vi "9.1.vi"() -> ()   [LabVIEW 2020]
panel:
  in  "module path 3":path=path "C:/Users/Oliver/Videos/ylesanne2.py"
  in  "Cluster":T1
  in  "Numeric 2":i32
  in  "Folat 2":dbl
  out "Waveform Graph":T1(graph)
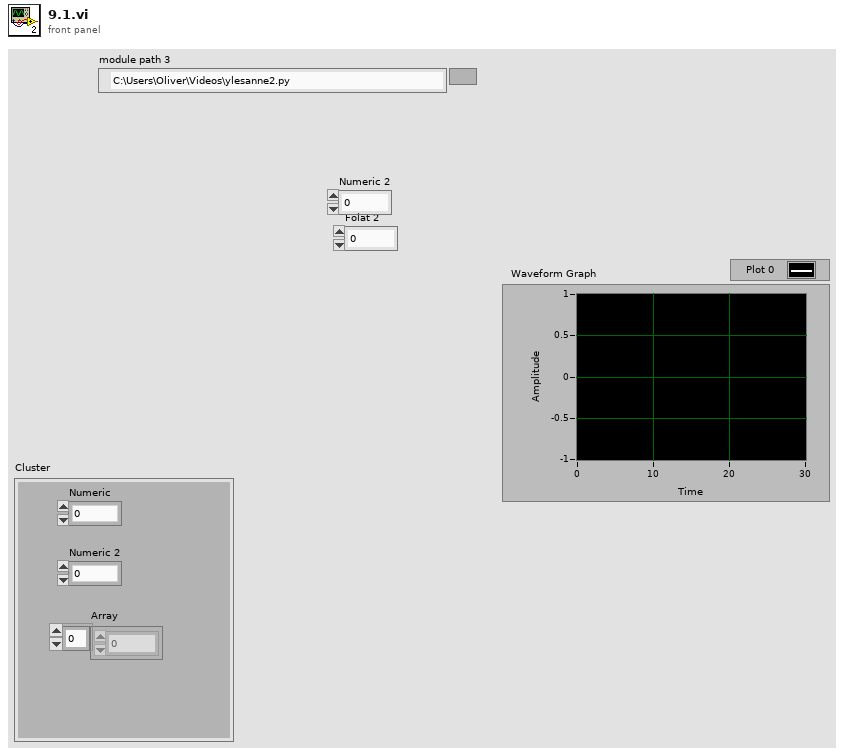
[diagram p1: front panel]
types:
  T1 = cluster{"Numeric":dbl, "Numeric 2":dbl, "Array":dbl[]}
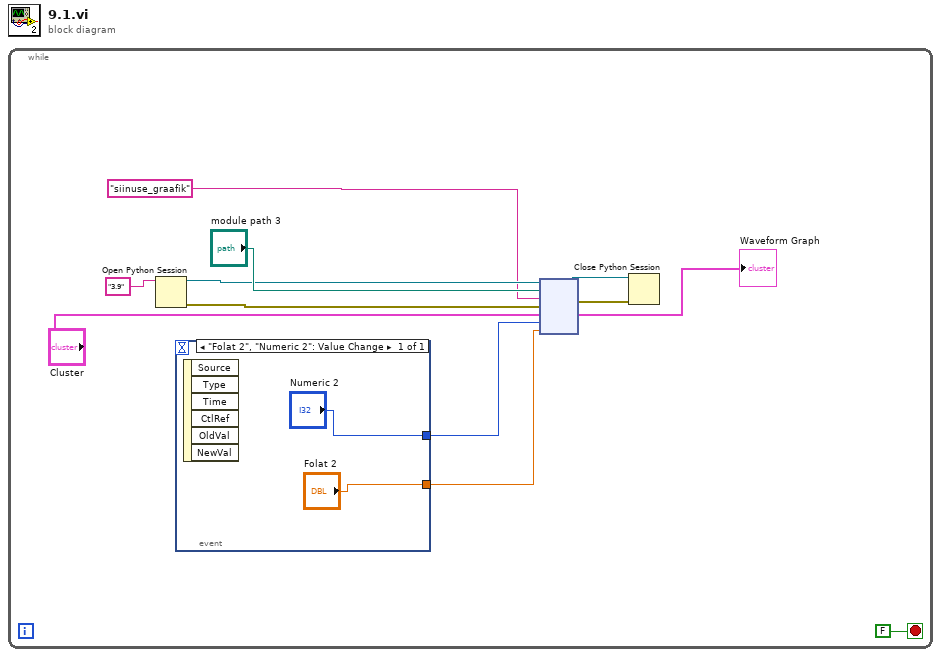
[diagram p0: block diagram]
diagram:
  n1 = while {
    stop <- FALSE stop-if-true
    n2 = Open Python Session(python version="3.9" ("Python version")) -> (session out=w10:refnum<k35>, error out=w9:errorcluster)  [unwired: 2 in]
    n3 = event shown="[0] \"Folat 2\", \"Numeric 2\": Value Change" {
      selector: _ -> [_]
      dyn-events: _ -> [_]
      timeout: _ -> [_]
      tunnel: ["Numeric 2"] -> w5
      tunnel: ["Folat 2"] -> w4
      event "Folat 2", "Numeric 2": Value Change {
        n4 = event-data() -> ()  [unwired: 1 in, 6 out]
      }
    }
    n5 = node(w10, "module path 3", "siinuse_graafik" ("function name"), w9, "Cluster", w5, w4) -> (w3:refnum<k35>, w2:errorcluster, →"Waveform Graph":T1)  [unwired: 2 in, 2 out]
    n6 = Close Python Session(session in=w3, error in=w2) -> ()  [unwired: 1 out]
  }
